vi "Load from LVTest File.vi"(8 "error in (no error)":errorcluster, 10 "LVTest File Path":path, 11 "LUnit Test Vector In":refnum<class "LUnit Test Vector.lvclass">) -> (0 "error out":errorcluster, 3 "LUnit Test Vector Out":refnum<class "LUnit Test Vector.lvclass">)   [LabVIEW 2020, in "LUnit Test Vector.lvclass"]
doc: "Loads tests from a file formated as a LVTest file and the content of the file is loaded into the test vector.\nThis method does not yet support all features used by the Unit Test Framework and the only comparison option which is accepted is \"=\"."
uses:
  LUnit Test Vector.lvclass
  LUnit Test Vector.lvclass/LUnit Test Vector.ctl
  <vilib>/ErrorRing/Error Ring.xnode
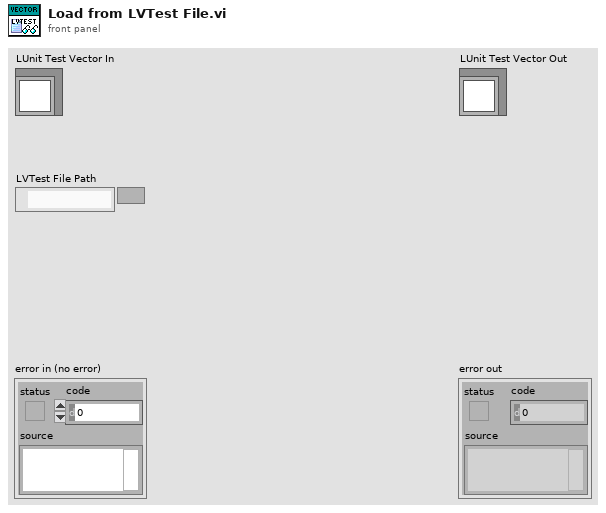
[diagram p1: front panel]
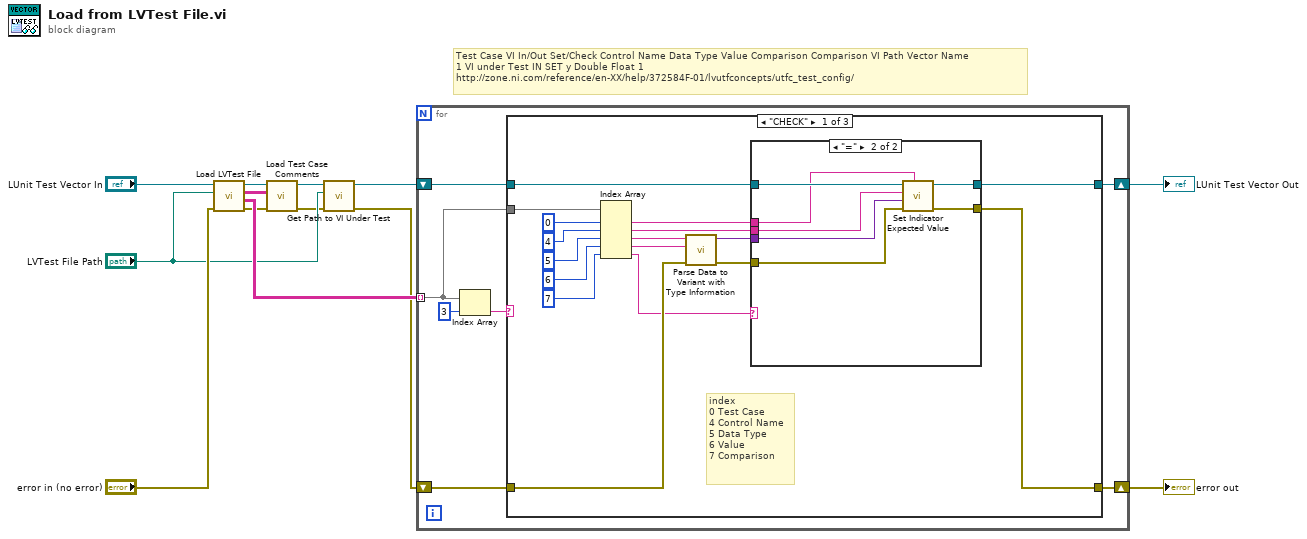
[diagram p0: block diagram]
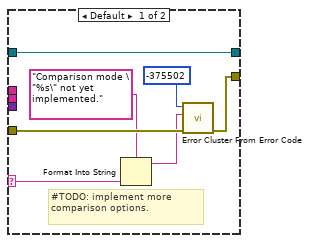
[diagram p2: hidden frame]
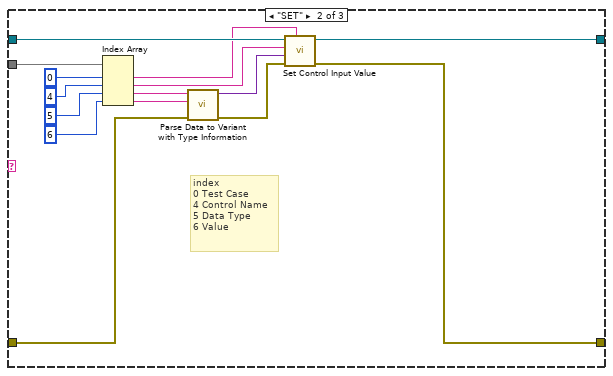
[diagram p3: hidden frame]
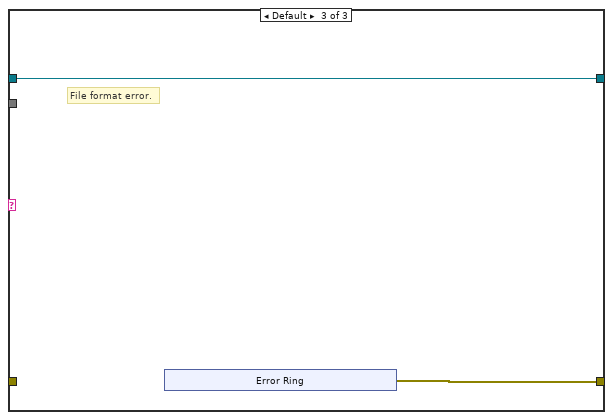
[diagram p4: hidden frame]
diagram:
  # "Test Case\tVI\tIn/Out\tSet/Check\tControl Name\tData Type\tValue\tComparison\tComparison VI Path\tVector Name\n1\tVI under Test\tIN\tSET\ty\tDouble Float\t1\t\t\t\nhttp://zone.ni.com/reference/en-XX/help/372584F-01/lvutfconcepts/utfc_test_config/"
  n1 = call "Load LVTest File.vi"("error in (no error)"="error in (no error)", "LVTest file"="LVTest File Path", "LUnit Test Vector In"="LUnit Test Vector In") -> ("error out"=w3:errorcluster, "Test Case Table"=w9:string[][], "File Contents"=w1:string[][], "LUnit Test Vector Out"=w5:refnum<class "LUnit Test Vector.lvclass">)  [unwired: 5 in]
  n2 = call "Load Test Case Comments.vi"("error in (no error)"=w3, "File Contents"=w1, "LUnit Test Vector In"=w5) -> ("error out"=w2:errorcluster, "LUnit Test Vector Out"=w4:refnum<class "LUnit Test Vector.lvclass">)  [unwired: 7 in]
  n3 = call "Get Path to VI Under Test.vi"("error in (no error)"=w2, "LVTest file"="LVTest File Path", "LUnit Test Vector in"=w4) -> ("error out"=w8:errorcluster, "LUnit Test Vector out"=w7:refnum<class "LUnit Test Vector.lvclass">)  [unwired: 7 in]
  n4 = for {
    tunnel: w9 -> [w16] mode=indexing
    shift-right: [w18] -> w11
    shift-left: w8 -> [w15]
    shift-right: [w14] -> w10
    shift-left: w7 -> [w17]
    n5 = Index Array(array=w16, index=3) -> (element=w19:string)
    n6 = case shown="\"CHECK\"" w19 {
      tunnel: [w31 w60 w68] -> w18
      tunnel: w17 -> [w37 w66 w67]
      tunnel: w16 -> [w35 w64 _]
      tunnel: w15 -> [w25 w54 _]
      tunnel: [w30 w59 w67] -> w14
      frame "CHECK" {
        # "index  \n0 Test Case \n4 Control Name\n5 Data Type \n6 Value\n7 Comparison"
        n7 = Index Array(array=w35, index #1=0 ("index"), index #2=4 ("index"), index #3=5 ("index"), index #4=6 ("index"), index #5=7 ("index")) -> (element #1=w34:string, element #2=w33:string, element #3=w27:string, element #4=w24:string, element #5=w21:string)
        n8 = call "Parse Data to Variant with Type Information.vi"("error in (no error)"=w25, "Data"=w24, "Datatype"=w27) -> ("error out"=w26:errorcluster, "Variant"=w23:variant)  [unwired: 7 in]
        n9 = case shown="\"=\"" w21 {
          selector: w21 -> [w39 _]
          tunnel: w37 -> [w44 w51]
          tunnel: w34 -> [_ w50]
          tunnel: w33 -> [_ w49]
          tunnel: [w43 w48] -> w31
          tunnel: [w44 w47] -> w30
          tunnel: w26 -> [w41 w46]
          tunnel: w23 -> [_ w45]
          frame Default {
            # "#TODO: implement more comparison options."
            n10 = Format Into String(format string="Comparison mode \"%s\" not yet implemented.", w39) -> (resulting string=w38:string)  [unwired: 2 in, 1 out]
            n11 = call <vilib>:"Error Cluster From Error Code.vi"("error in (no error)"=w41, "error message (\"\")"=w38, "error code (0)"=-375502) -> ("error out"=w43:errorcluster)  [unwired: 6 in]
          }
          frame "=" {
            n12 = call "Set Indicator Expected Value.vi"("Vector Component"=w50, "error in (no error)"=w46, "Data"=w45, "Control Name"=w49, "LUnit Test Vector In"=w51) -> ("error out"=w48:errorcluster, "LUnit Test Vector Out"=w47:refnum<class "LUnit Test Vector.lvclass">)  [unwired: 5 in]
          }
        }
      }
      frame "SET" {
        # "index  \n0 Test Case \n4 Control Name\n5 Data Type \n6 Value"
        n13 = Index Array(array=w64, index #1=0 ("index"), index #2=4 ("index"), index #3=5 ("index"), index #4=6 ("index")) -> (element #1=w63:string, element #2=w62:string, element #3=w56:string, element #4=w53:string)
        n14 = call "Parse Data to Variant with Type Information.vi"("error in (no error)"=w54, "Data"=w53, "Datatype"=w56) -> ("error out"=w55:errorcluster, "Variant"=w52:variant)  [unwired: 7 in]
        n15 = call "Set Control Input Value.vi"("Vector Component"=w63, "error in (no error)"=w55, "Data"=w52, "Control Name"=w62, "LUnit Test Vector In"=w66) -> ("error out"=w60:errorcluster, "LUnit Test Vector Out"=w59:refnum<class "LUnit Test Vector.lvclass">)  [unwired: 5 in]
      }
      frame Default {
        # "File format error."
        n16 = xnode "Error Ring"() -> ("error out"=w68:errorcluster)
      }
    }
  }
  "error out" <- w11
  "LUnit Test Vector Out" <- w10
